vi "IMAQdx_setAttribute_Enum.vi"(4 "error in (no error)":errorcluster, 5 "Value (Enum)":u32(ring), 6 "Attribute Name":string, 7 "IMAQdx Session":T1) -> (0 "error out":errorcluster, 1 "In Range?":bool, 3 "dup IMAQdx Session":T1)   [LabVIEW 2014, in "HGF_VisionTools.lvlib"]
doc: "This VI sets IMAQdx attribute value of type enumeration."
uses:
  HGF_VisionTools.lvlib
  <resource>/objmgr/imaqdx.rc
  HGF_LVC/HGF_Auxiliary/HGF_Auxiliary.lvlib
  HGF_LVC/HGF_Auxiliary/Severity.ctl
  HGF_LVC/HGF_Auxiliary/ErrorCode.ctl
  <vilib>/userdefined/High Color/IMAQdx.ctl
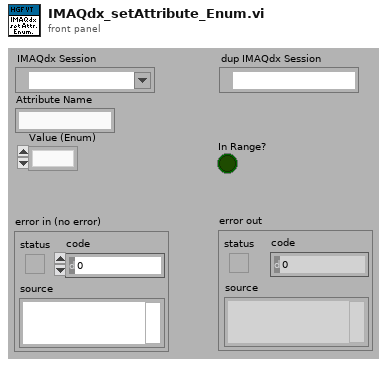
[diagram p1: front panel]
types:
  T1 = typedef "IMAQdx.ctl" = refnum<k21>
  T2 = typedef "HGF_Auxiliary.lvlib/ErrorCode.ctl" = enum32{"No error", "Function not supported.", "This VI is for friends only.", "Reference object aready exisits.", "Parameter out of range.", "Not a rendezvous.", "Invalid notifier reference.", "Invalid queue reference.", "Self-Test not supported.", "Reset not supported.", "IDN query not supported.", "Error query not supported.", "Incorrect addressee.", "Object already exists.", "No class name specified", "Driver not supported", "Attribute is not writable"}
  T3 = typedef "HGF_Auxiliary.lvlib/Severity.ctl" = enum16{"Info", "Warning", "Fault", "Error", "Fatal"}
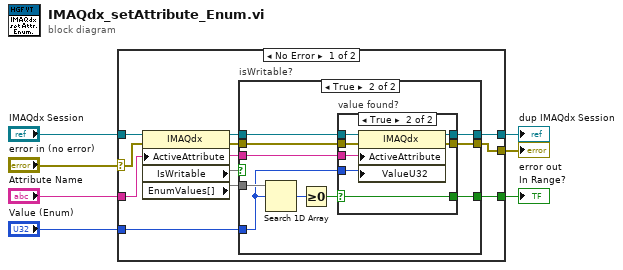
[diagram p0: block diagram]
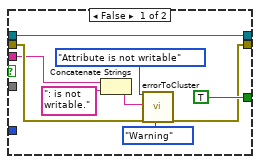
[diagram p2: hidden frame]
diagram:
  n1 = case shown="No Error" "error in (no error)" {
    selector: "error in (no error)" -> [w9 w48]
    tunnel: "IMAQdx Session" -> [w18 w49]
    tunnel: "Attribute Name" -> [w15 _]
    tunnel: "Value (Enum)" -> [w13 _]
    tunnel: [w12 w49] -> w4
    tunnel: [w11 w48] -> w3
    tunnel: [w10 _] -> w2
    frame No Error {
      n2 = property class="IMAQdx"(reference=w18, error in=w9, "ActiveAttribute"=w15) -> (reference out=w17:T1, error out=w16:errorcluster, "IsWritable"=w8, "EnumValues[]"=w14)
      n3 = case "isWritable?" shown="True" w8 {
        tunnel: w17 -> [w27 w37]
        tunnel: w16 -> [w21 w36]
        tunnel: w15 -> [w20 w35]
        tunnel: w14 -> [_ w32]
        tunnel: w13 -> [_ w31]
        tunnel: [w27 w34] -> w12
        tunnel: [w19 w33] -> w11
        tunnel: [TRUE w28] -> w10
        frame False {
          n4 = Concatenate Strings(w20, ": is not writable." ("string")) -> (w22:string)
          n5 = call "errorToCluster.vi"("error code"=ErrorCode."Attribute is not writable", "error message (\"\")"=w22, "error in (no error)"=w21, "severity (Error)"=Severity."Warning") -> ("error out"=w19:errorcluster)  [unwired: 15 in]
        }
        frame True {
          n6 = Search 1D Array(1D array=w32, element=w31) -> (index of element=w30:i32)  [unwired: 1 in]
          n7 = Greater Or Equal To 0?(x=w30) -> (x >= 0?=w29:bool)
          n8 = case "value found?" shown="True" w29 {
            selector: w29 -> [w40 w41]
            tunnel: w37 -> [w39 w47]
            tunnel: w36 -> [w38 w46]
            tunnel: w35 -> [_ w45]
            tunnel: [w39 w44] -> w34
            tunnel: [w38 w43] -> w33
            tunnel: w31 -> [_ w42]
            tunnel: [w40 w41] -> w28
            frame False {
            }
            frame True {
              n9 = property class="IMAQdx"(reference=w47, error in=w46, "ActiveAttribute"=w45, "ValueU32"=w42) -> (reference out=w44:T1, error out=w43:errorcluster)
            }
          }
        }
      }
    }
    frame Error {
    }
  }
  "dup IMAQdx Session" <- w4
  "error out" <- w3
  "In Range?" <- w2
